vi "PH_Beckhoff_PP_PU.evt Call Ignitron on.vi"(0 "i ref in":refnum<vi>, 3 "PU":T1, 5 "error in":errorcluster) -> (14 "i ref out":refnum<vi>, 19 "error out":errorcluster)   [LabVIEW 2014, in "PH_Beckhoff_PP_PU.lvlib"]
doc: "This VI calls an event by a simple call."
uses:
  PH_Beckhoff_PP_PU.lvlib
  PH_PP_Common/PH_PP_Common.PUs.ctl
  PH_Beckhoff_PP_PU.Igni Tags.ctl
  PH_Beckhoff/PH_Beckhoff.lvlib
  PH_PP_Common/PH_PP_Common.lvlib
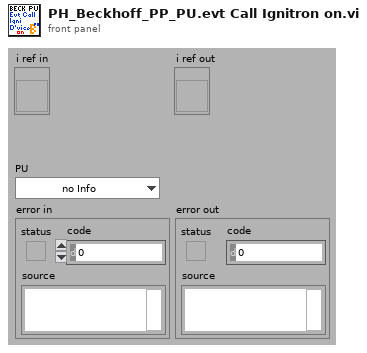
[diagram p1: front panel]
types:
  T1 = typedef "PH_PP_Common.lvlib/PH_PP_Common.PUs.ctl" = enum16{"no Info", "PA-19mm-1", "PA-19mm-2", "PA-45mm-PILC", "PA-45mm-MAIN", "MA-PU-1", "MA-PU-2", "MA-PU-3", "MA-PU-4", "MA-PU-5", "MA-PU-6", "MA-FR", "MA-PILC", "PA-45mm-DP"}
  T2 = typedef "PH_Beckhoff_PP_PU.lvlib/PH_Beckhoff_PP_PU.Igni Tags.ctl" = enum16{"heating-on", "water-on", "Device-on", "Status"}
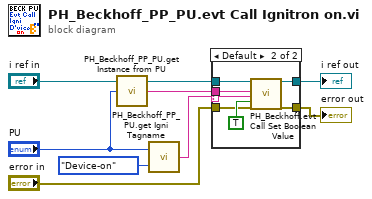
[diagram p0: block diagram]
diagram:
  n1 = call "PH_Beckhoff_PP_PU.get Instance from PU.vi"("PU"="PU") -> ("Beckhoff PU Instance"=w2:string)
  n2 = call "PH_Beckhoff_PP_PU.get Igni Tagname.vi"("Igni Tag"=PH_Beckhoff_PP_PU.Igni_Tags."Device-on", "PU"="PU") -> ("Igni Tagname"=w4:string)
  n3 = case shown="Default" w4 {
    selector: w4 -> [_ w11]
    tunnel: [w9 w17] -> w8
    tunnel: w2 -> [_ w15]
    tunnel: "error in" -> [w9 w14]
    tunnel: [w10 w13] -> w6
    tunnel: "i ref in" -> [w10 w12]
    frame "", "N/A" {
    }
    frame Default {
      n4 = call "PH_Beckhoff.evt Call Set Boolean Value.vi"("i ref in"=w12, "Beckhoff Instance"=w15, "Tagname to set"=w11, "Value"=TRUE ("NewVal"), "error in"=w14) -> ("i ref out"=w13:refnum<vi>, "error out"=w17:errorcluster)  [unwired: 13 in]
    }
  }
  "error out" <- w8
  "i ref out" <- w6
